vi "se1e2.vi"() -> ()   [LabVIEW 2013]
panel:
  out "Numeric":dbl
  out "Boolean":bool
  out "A-B":dbl
  out "A+B":dbl
  in  "B":dbl
  in  "A":dbl
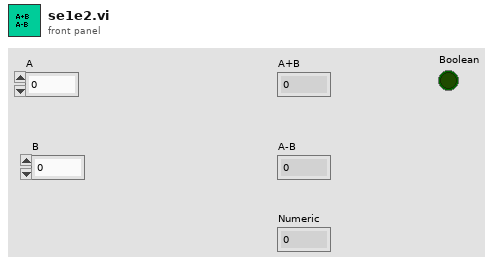
[diagram p1: front panel]
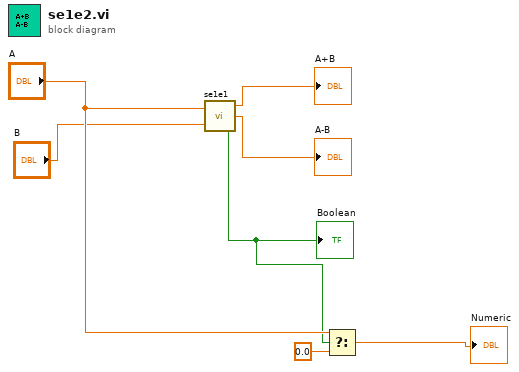
[diagram p0: block diagram]
diagram:
  n1 = call "se1e1.vi"("A"="A", "B"="B") -> ("Numeric 2"=→"A+B":dbl, "Numeric"=→"A-B":dbl, "x = y?"=w1:bool)
  "Boolean" <- w1
  n2 = Select(t="A", s=w1, f=0.0) -> (s? t:f=→"Numeric":dbl)
